vi "Read Test Case object from front panel control.vi"(8 "error in (no error)":errorcluster, 10 "VI Refnum":refnum<vi>, 11 "Test Case in":refnum<class "LUnit Test Case.lvclass">) -> (0 "error out":errorcluster, 2 "VI Refnum out":refnum<vi>, 3 "Test Case out":refnum<class "LUnit Test Case.lvclass">)   [LabVIEW 2020, in "Slave Test Runner.lvclass"]
uses:
  Slave Test Runner.lvclass
  Test Case/LUnit Test Case.lvclass
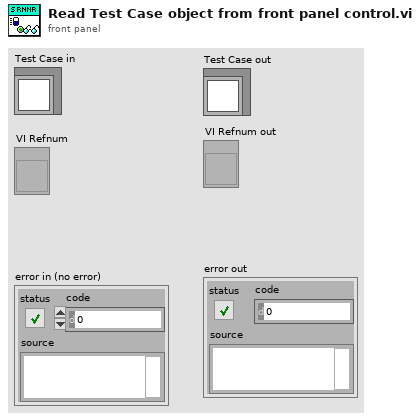
[diagram p1: front panel]
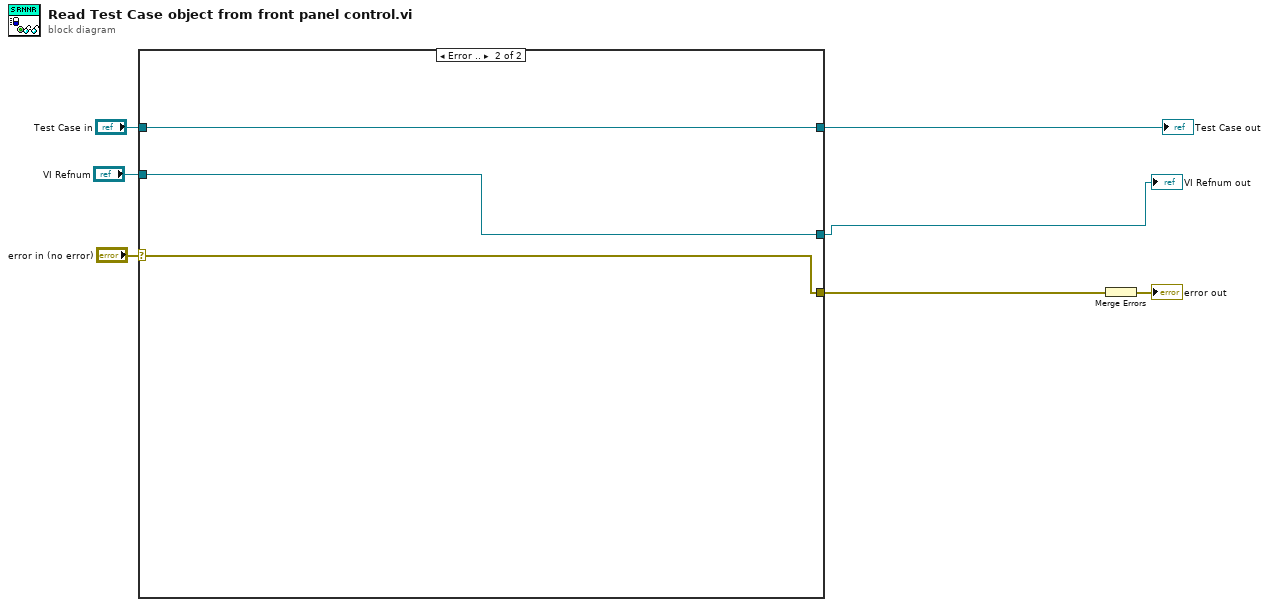
[diagram p0: block diagram]
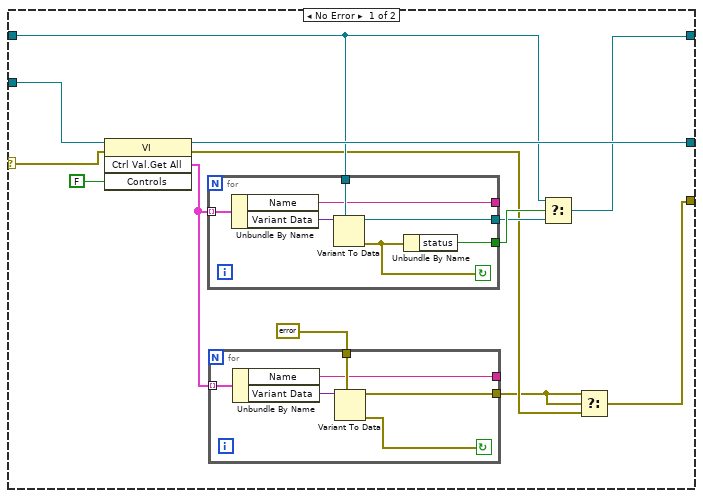
[diagram p2: hidden frame]
diagram:
  n1 = case shown="Error .." "error in (no error)" {
    selector: "error in (no error)" -> [w20 w35]
    tunnel: "VI Refnum" -> [w18 w36]
    tunnel: [w17 w36] -> w1
    tunnel: [w9 w35] -> w2
    tunnel: [w16 w34] -> w5
    tunnel: "Test Case in" -> [w13 w34]
    frame No Error {
      n2 = invoke on="Invoke Node" class="VI" method="Ctrl Val.Get All"(reference=w18, error in=w20, "Controls"=FALSE) -> (reference out=w17:refnum<vi>, error out=w10:errorcluster, "Get All Control Values Variant"=w12:cluster{"Name":string, "Variant Data":variant}[])  [unwired: 1 in, 1 out]
      n3 = for {
        tunnel: w12 -> [w33] mode=indexing
        tunnel: w13 -> [w31]
        tunnel: [w30] -> _
        tunnel: [w28] -> w15
        tunnel: [w27] -> w14
        stop <- w29 continue-if-true
        n4 = Unbundle By Name(w33) -> ("Name"=w30:string, "Variant Data"=w32:variant)
        n5 = Variant To Data(type=w31, Variant=w32) -> (data=w27:refnum<class "LUnit Test Case.lvclass">, error out=w29:errorcluster)  [unwired: 1 in]
        n6 = Unbundle By Name(w29) -> ("status"=w28:bool)
      }
      n7 = for {
        tunnel: w12 -> [w26] mode=indexing
        tunnel: errorcluster {"status"=FALSE, "code"=0, "source"=""} ("error IO") -> [w24]
        tunnel: [w23] -> _
        tunnel: [w21] -> w8
        stop <- w22 continue-if-true
        n8 = Unbundle By Name(w26) -> ("Name"=w23:string, "Variant Data"=w25:variant)
        n9 = Variant To Data(type=w24, Variant=w25) -> (data=w21:errorcluster, error out=w22:errorcluster)  [unwired: 1 in]
      }
      n10 = Select(t=w13, s=w15, f=w14) -> (s? t:f=w16:refnum<class "LUnit Test Case.lvclass">)
      n11 = Select(t=w8, s=w8, f=w10) -> (s? t:f=w9:errorcluster)
    }
    frame Error {
    }
  }
  "VI Refnum out" <- w1
  "Test Case out" <- w5
  n12 = Merge Errors(w2) -> (→"error out":errorcluster)
